vi "RFController getDPDKKPIStream Read.vi"(8 "error in":errorcluster, 11 "Call ID in":T3) -> (0 "error out":errorcluster, 1 "Success":bool, 2 "Response Data":T1, 3 "Call ID":T3)   [LabVIEW 2024, in "FlexCompute_grpc_client.lvlib"]
uses:
  FlexCompute_grpc_client.lvlib
  <vilib>/gRPC/LabVIEW gRPC Library/Shared/grpcId.ctl
  RPC Messages/rfcontrol_KPIData.ctl
  RPC Messages/rfcontrol_Status.ctl
  RPC Messages/rfcontrol_KPIData_Flat.ctl
  aea5dbbb-03a2-479b-ad95-94da4ee1cea9.vi
  <vilib>/gRPC/LabVIEW gRPC Library/Shared/TranslateGrpcError.vi
  <vilib>/gRPC/LabVIEW gRPC Library/Shared/Wait On Occurrence.vi
  <vilib>/gRPC/LabVIEW gRPC Library/Shared/Is Feature Enabled.vi
  <vilib>/gRPC/LabVIEW gRPC Library/Server API/Server/Get Server DLL Path.vi
  <vilib>/Utility/error.llb/Error Cluster From Error Code.vi
  <vilib>/gRPC/LabVIEW gRPC Library/grpc-lvsupport-release.lvlib
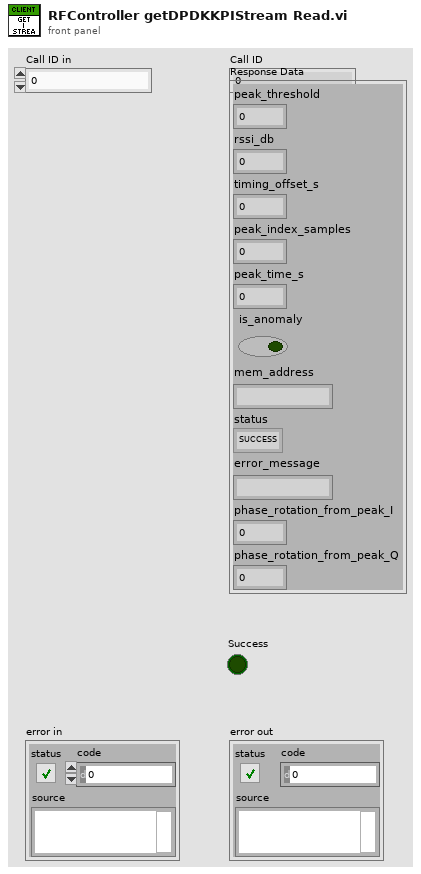
[diagram p1: front panel]
types:
  T1 = typedef "FlexCompute_grpc_client.lvlib/rfcontrol_KPIData.ctl" = cluster{"peak_threshold":dbl, "rssi_db":dbl, "timing_offset_s":dbl, "peak_index_samples":i32, "peak_time_s":dbl, "is_anomaly":bool, "mem_address":string, "status":T2, "error_message":string, "phase_rotation_from_peak_I":sgl, "phase_rotation_from_peak_Q":sgl}
  T2 = typedef "FlexCompute_grpc_client.lvlib/rfcontrol_Status.ctl" = enum32{"SUCCESS", "ERROR"}
  T3 = typedef "grpc-lvsupport-release.lvlib/grpcId.ctl" = u64
  T4 = typedef "FlexCompute_grpc_client.lvlib/rfcontrol_KPIData_Flat.ctl" = cluster{"peak_threshold":dbl, "rssi_db":dbl, "timing_offset_s":dbl, "peak_index_samples":i32, "peak_time_s":dbl, "is_anomaly":bool, "mem_address":string, "status":T2, "error_message":string, "phase_rotation_from_peak_I":sgl, "phase_rotation_from_peak_Q":sgl}
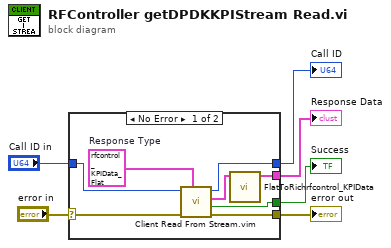
[diagram p0: block diagram]
diagram:
  n1 = case shown="No Error" "error in" {
    selector: "error in" -> [w14 w15]
    tunnel: [w13 w15] -> w5
    tunnel: "Call ID in" -> [w12 w16]
    tunnel: [w10 w16] -> w3
    tunnel: [w7 _] -> w2
    tunnel: [w11 _] -> w1
    frame No Error {
      w9 = T4 {"peak_threshold"=0.0, "rssi_db"=0.0, "timing_offset_s"=0.0, "peak_index_samples"=0, "peak_time_s"=0.0, "is_anomaly"=FALSE, "mem_address"="", "status"=enum."SUCCESS", "error_message"="", "phase_rotation_from_peak_I"=0.0, "phase_rotation_from_peak_Q"=0.0}  # Response Type
      n2 = call "Client Read From Stream.vim"("Response Type"=w9, "error in"=w14, "Call ID in"=w12) -> ("error out"=w13:errorcluster, "Success"=w11:bool, "Response Data"=w8:T4, "Call ID out"=w10:u64)  [unwired: 5 in]
      n3 = call "FlatToRichrfcontrol_KPIData.vi"("InputCluster"=w8) -> ("OutputCluster"=w7:T1)  [unwired: 10 in]
    }
    frame Error {
    }
  }
  "error out" <- w5
  "Call ID" <- w3
  "Response Data" <- w2
  "Success" <- w1
